vi "test13-AsteriskWildcardStateRegistration.vi"(8 "error in (no error)":errorcluster, 11 "TestCase in":refnum<class "testcase-CSMBroadcast.lvclass">) -> (0 "error out":errorcluster, 3 "TestCase out":refnum<class "testcase-CSMBroadcast.lvclass">)   [LabVIEW 2017, in "testcase-CSMBroadcast.lvclass"]
uses:
  testcase-CSMBroadcast.lvclass
  0c20cacf-7d77-4f8e-aec5-f22e7d09936d.vi
  26de337d-8090-412f-9da5-e117a55d4726.vi
  de10340a-d592-45ad-b055-7fa7b377c551.vi
  e3eae2f8-d8ce-4adb-8167-9a417250fce1.vi
  a4d00e00-a9ed-4631-bf53-269bf71f16fc.vi
  src/user.lib/_NEVSTOP/Communicable State Machine(CSM)/AdvanceAPI/CSM - Revert Arguments-Safe String.vi
  src/user.lib/_NEVSTOP/Communicable State Machine(CSM)/_Shared/Trim Single-line Text.vi
  src/user.lib/_NEVSTOP/Communicable State Machine(CSM)/AdvanceAPI/CSM - Make String Arguments Safe.vi
  src/user.lib/_NEVSTOP/Communicable State Machine(CSM)/AdvanceAPI/CSM - Break Down Multiple States String.vi
  src/user.lib/_NEVSTOP/Communicable State Machine(CSM)/AdvanceAPI/CSM - Compact Multiple States.vi
  src/user.lib/_NEVSTOP/Communicable State Machine(CSM)/AdvanceAPI/CSM - Keywords.vi
  src/user.lib/_NEVSTOP/Communicable State Machine(CSM)/AdvanceAPI/CSM - Set Module Attribute.vi
  src/user.lib/_NEVSTOP/Communicable State Machine(CSM)/AdvanceAPI/CSM - Get Module Attribute.vi
  <vilib>/addons/_JKI Toolkits/VI Tester/TestCase.llb/TestCase.lvclass
  src/user.lib/_NEVSTOP/Communicable State Machine(CSM)/Communicable State Machine.lvlib
  C:/Program Files (x86)/National Instruments/LabVIEW 2017/vi.lib/addons/_JKI Toolkits/VI Tester/TestCase.llb/TestCase.lvclass
panel:
  out "Execution Times":i32
  out "State History":string
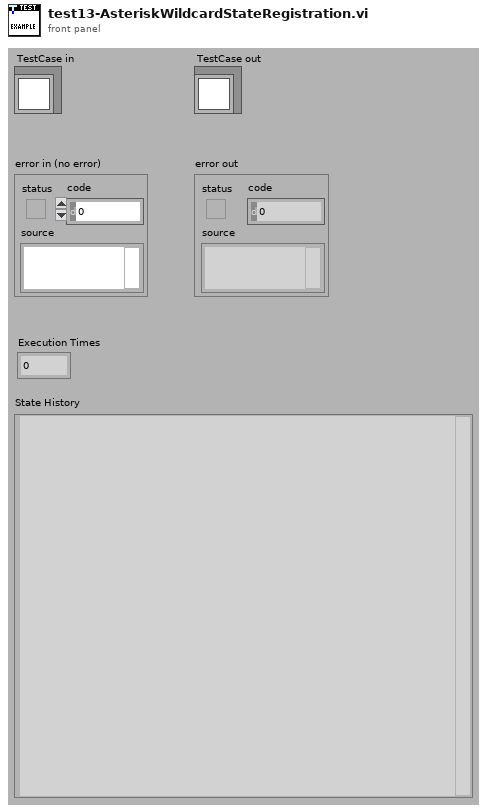
[diagram p1: front panel]
types:
  T1 = enum32{"Invalid", "Standard", "Closed", "Hidden", "Minimized", "Maximized"}
  T2 = enum32{"invalid app kind", "Development System", "Run Time System", "Student Edition", "Embedded LabVIEW", "Evaluation", "Custom"}
  T3 = typedef "Communicable State Machine.lvlib/_CSM_Response Source Message.ctl" = cluster{"‘State":string, "’Arguments":string, "’Error":errorcluster}
  T4 = cluster{"Current VI Reference":refnum<vi>, "Close Panel on Exit?":bool}
  T5 = cluster{"Core":cluster{"Current VI Reference":refnum<vi>, "Close Panel on Exit?":bool}, "Your Boolean data":bool, "Your string data":string, "TestData":i32}
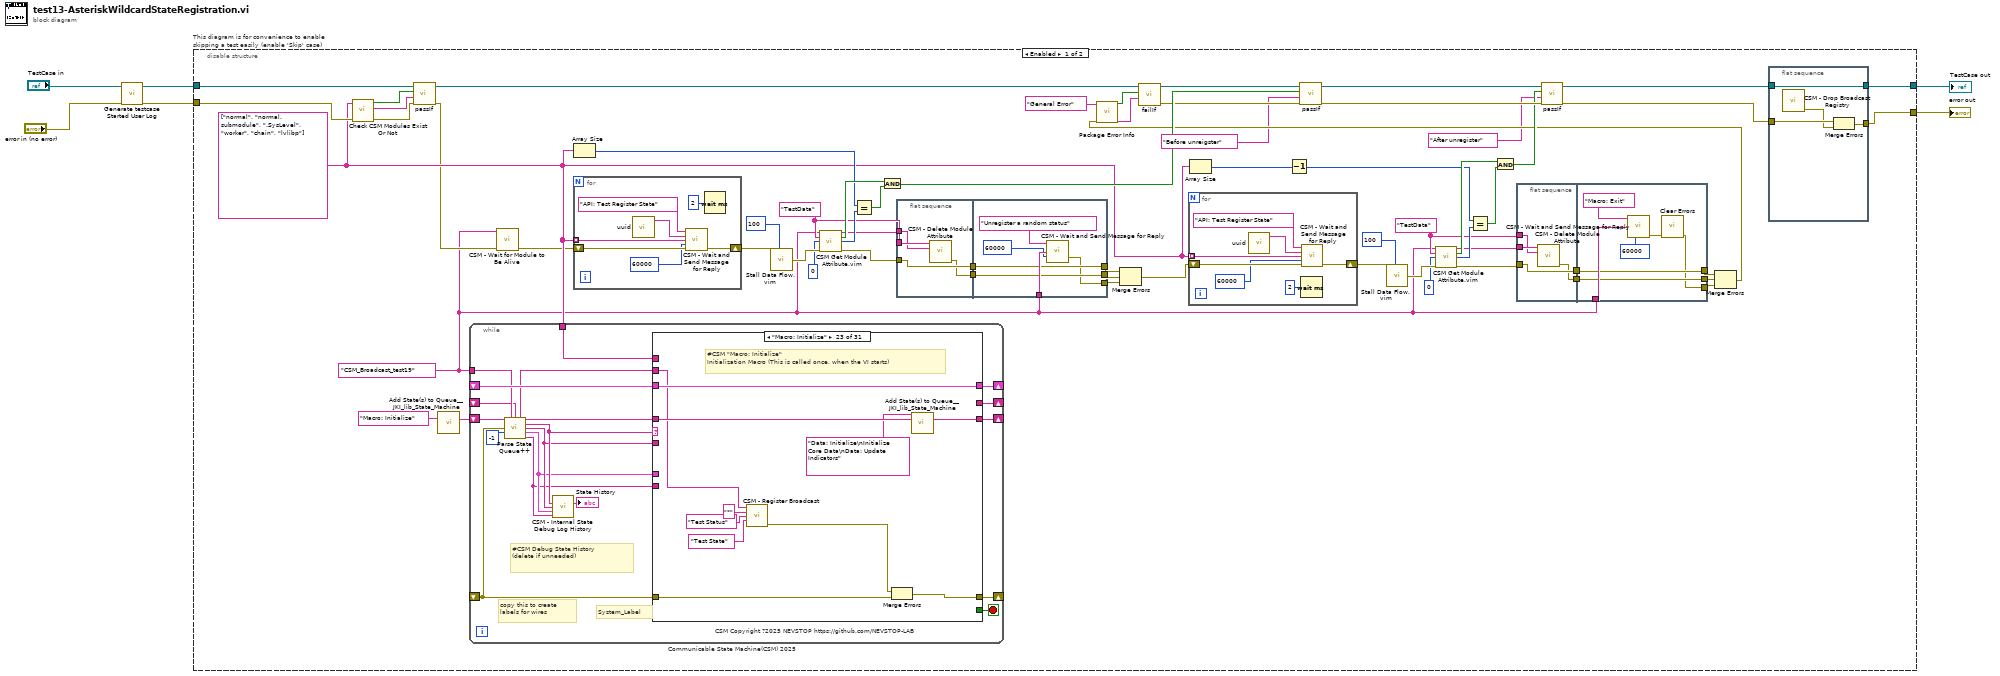
[diagram p0: block diagram]
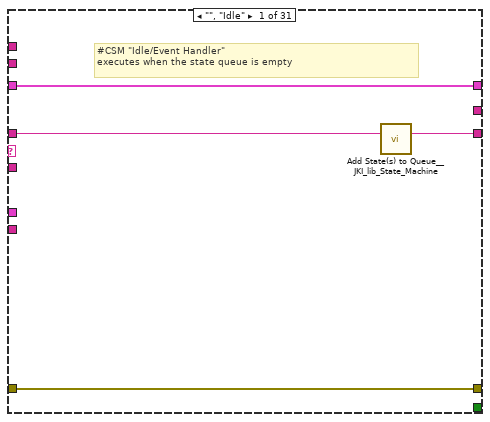
[diagram p2: hidden frame]
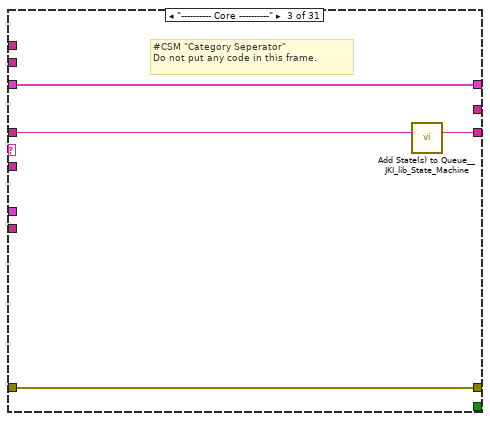
[diagram p4: hidden frame]
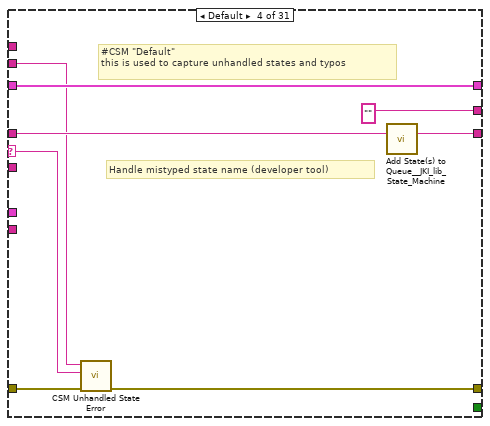
[diagram p5: hidden frame]
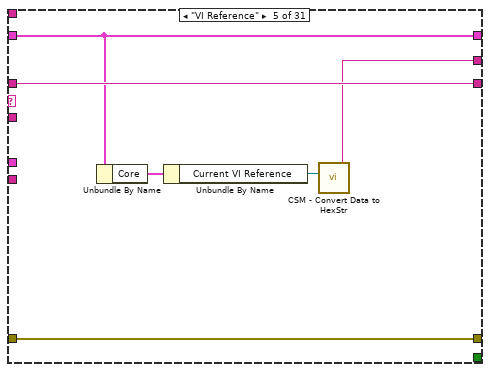
[diagram p6: hidden frame]
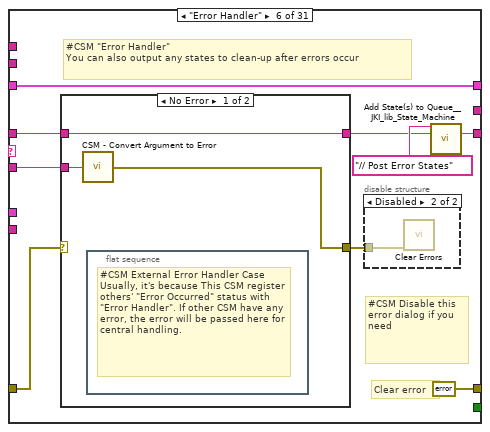
[diagram p7: hidden frame]
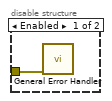
[diagram p8: hidden frame]
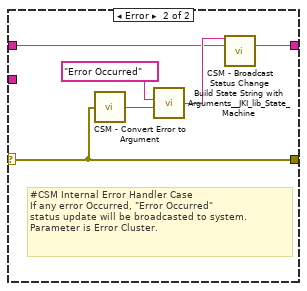
[diagram p9: hidden frame]
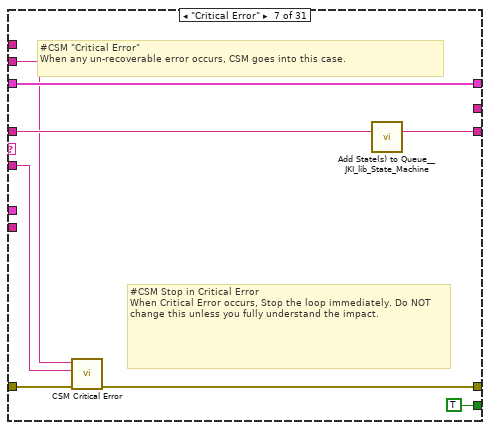
[diagram p10: hidden frame]
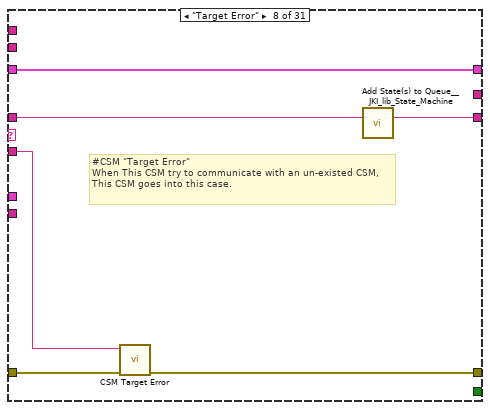
[diagram p11: hidden frame]
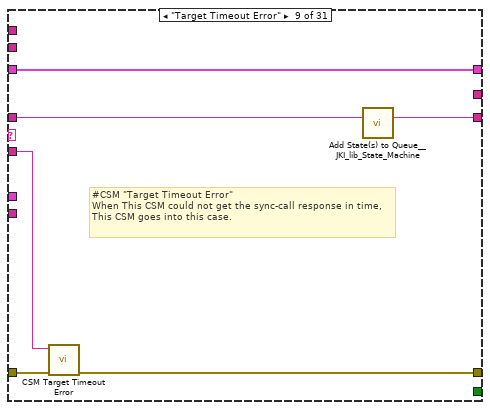
[diagram p12: hidden frame]
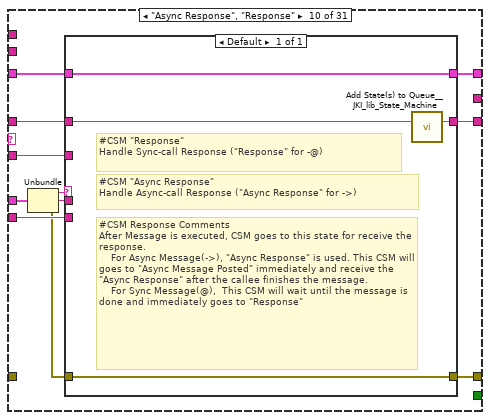
[diagram p13: hidden frame]
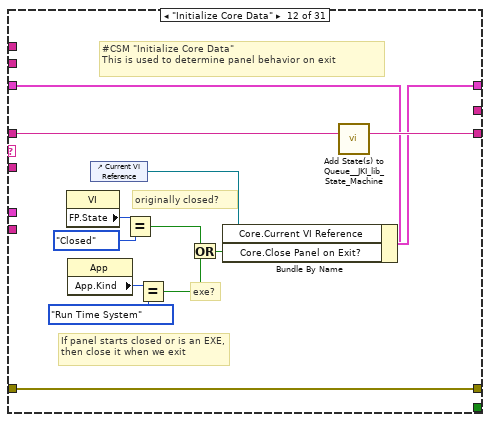
[diagram p15: hidden frame]
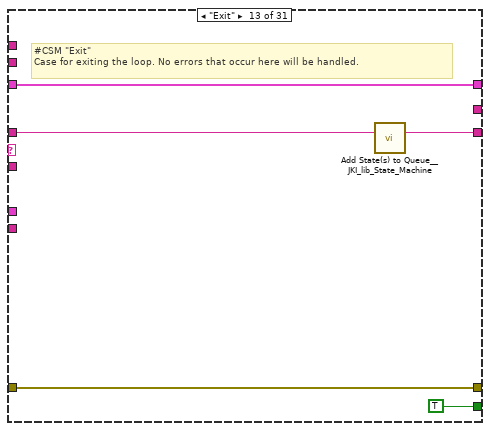
[diagram p16: hidden frame]
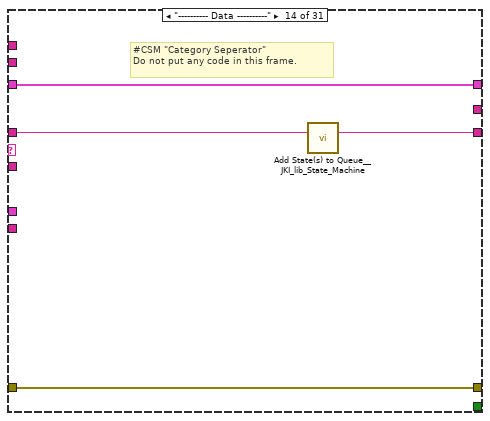
[diagram p17: hidden frame]
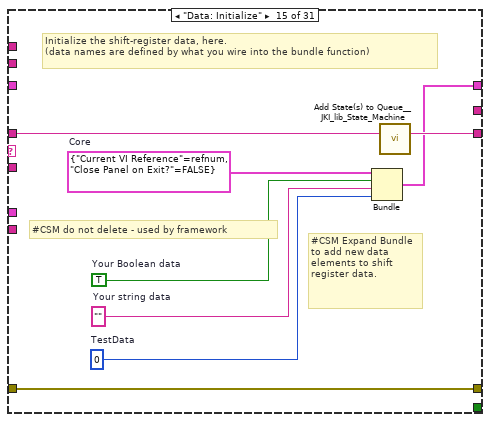
[diagram p18: hidden frame]
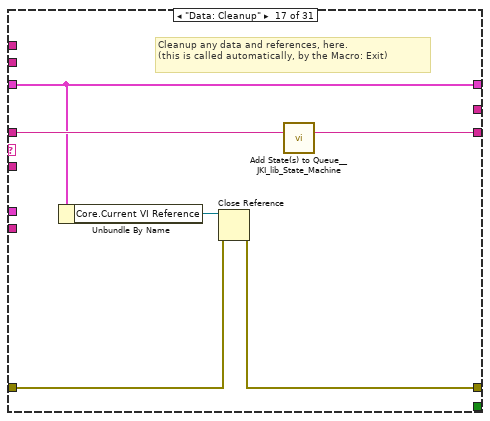
[diagram p20: hidden frame]
diagram:
  n1 = call "Generate testcase Started User Log.vi"("Error In"="error in (no error)") -> ("error out"=w1:errorcluster)  [unwired: 10 in]
  n2 = disable-structure "This diagram is for convenience to enable skipping a test easily (enable 'Skip' case)" shown="Enabled" {
    disable-tunnel: "TestCase in" -> [w24 w426]
    disable-tunnel: [w19 w424] -> w2
    disable-tunnel: [w18 w425] -> w4
    disable-tunnel: w1 -> [w23 w423]
    frame Enabled {
      w33 = "TestData" ("Attribute")
      w55 = "TestData" ("Attribute")
      w6 = "CSM_Broadcast_test19" ("Name (\"\" to Use UUID)")
      w22 = string[] ["normal", "normal.submodule", ".SysLevel", "worker", "chain", "lvlibp"]
      n3 = call "Check CSM Modules Exist Or Not.vi"("error in"=w23, "CSM names in"=w22) -> ("error out"=w25:errorcluster, "Debug string"=w26:string, "All Modules Exist?"=w27:bool)  [unwired: 7 in]
      n4 = call-dynamic "passIf.vi"("error in (no error)"=w25, "message (\"\")"=w26, "pass"=w27, "TestCase in"=w24) -> ("error out"=w7:errorcluster, "TestCase out"=w16:refnum<class "testcase-CSMBroadcast.lvclass">)  [unwired: 6 in]
      n5 = call <vilib>:"Add State(s) to Queue__JKI_lib_State_Machine.vi"("State(s) in (\"\")"="Macro: Initialize" ("Init State(\"Macro: Initialize\")")) -> ("States Out"=w66:string)  [unwired: 14 in]
      n6 = while "Communicable State Machine(CSM) 2025" {
        shift-right: [w113] -> _
        shift-left: _ -> [w112]
        shift-right: [w116] -> _
        shift-left: _ -> [w111]
        shift-right: [w115] -> _
        shift-left: w66 -> [w117]
        tunnel: w6 -> [w109]
        shift-right: [w110] -> _
        shift-left: _ -> [w103]
        tunnel: w22 -> [w100]
        stop <- w114 stop-if-true
        # "#CSM Debug State History\n(delete if unneeded)"
        # "copy this to create labels for wires"
        # "System_Label"
        # "CSM Copyright ?2025 NEVSTOP https://github.com/NEVSTOP-LAB"
        n7 = call "Parse State Queue++.vi"("State Queue"=w117, "Name (\"\" to Use UUID)"=w109, "Response Arguments"=w103, "Previous Error"=w111, "Dequeue (1 ms)"=-1 ("Timeout")) -> ("Name Used"=w104:string, "Remaining States"=w118:string, "Current State"=w108:string, "Arguments"=w107:string, "Additional Information"=w106:T3, "Source CSM"=w105:string)  [unwired: 5 in]
        n8 = call "CSM - Internal State Debug Log History.vi"("State"=w108, "Arguments (\"\")"=w107, ">> Response Source Message >>"=w106, "Source (\"\")"=w105) -> ("Debug Log"=→"State History":string)  [unwired: 11 in]
        n9 = case shown="\"Macro: Initialize\"" w108 {
          selector: w108 -> [_ _ _ w132 _ _ _ _ _ _ _ _ _ _ _ _ _ _ _ _ _ _ _ _ _ _ _ _ _ _ _]
          tunnel: w118 -> [w119 w124 w129 w136 w142 w148 w169 w175 w181 w189 w200 w214 w219 w223 w231 w233 w240 w244 w248 w254 w269 w338 w349 w362 w364 w368 w373 w380 w384 w395 w415]
          tunnel: w107 -> [_ _ _ _ _ w147 w165 w174 w179 w188 _ _ _ _ _ _ _ _ _ w249 w263 _ _ _ _ _ w371 _ _ _ _]
          tunnel: w112 -> [w120 w123 w126 w134 w141 w151 w170 w176 w182 w191 w199 w207 w217 w220 _ w232 w235 w241 w246 w252 w265 w335 w346 w359 w363 w367 w372 w377 w381 w387 w401]
          tunnel: [w121 w125 w127 w130 w143 errorcluster {"status"=FALSE, "code"=0, "source"=""} ("error out") w166 w172 w178 w194 w201 w211 w216 w221 w228 w234 w236 w242 w245 w250 w266 w336 w340 w351 w365 w369 w374 w378 w382 w389 w403] -> w116
          tunnel: w111 -> [w121 w125 w127 w137 w143 w149 w171 w173 w180 _ w201 w211 w216 w221 w228 w234 w237 w242 w245 w251 w267 w336 w347 w360 w365 w369 w374 w378 w382 w393 w413]
          tunnel: [w122 w124 w128 w135 w142 w144 w168 w177 w183 w190 w200 w213 w218 w222 w230 w233 w239 w243 w247 w253 w268 w337 w348 w361 w364 w368 w373 w379 w383 w394 w414] -> w115
          tunnel: [_ _ _ _ _ _ TRUE _ _ _ _ _ TRUE _ _ _ _ _ _ _ _ _ _ _ _ _ _ _ _ _ _] -> w114
          tunnel: [w120 w123 w126 w134 w141 w151 w170 w176 w182 w192 w199 w212 w217 w220 w229 w232 w235 w241 w246 w252 w265 w335 w346 w359 w363 w367 w372 w377 w381 w391 w399] -> w113
          tunnel: w105 -> [_ _ _ _ _ _ _ _ _ w186 _ _ _ _ _ _ _ _ _ _ _ _ _ _ _ _ _ _ _ _ _]
          tunnel: w106 -> [_ _ _ _ _ _ _ _ _ w193 _ _ _ _ _ _ _ _ _ _ _ _ _ _ _ _ _ _ _ _ _]
          tunnel: [_ _ _ "" w138 _ _ _ _ _ _ _ _ _ _ _ _ _ _ _ _ _ _ _ _ "API1 Response" w370 _ _ _ _] -> w110
          tunnel: w104 -> [_ _ _ w131 _ _ w164 _ _ _ _ _ _ _ _ _ _ _ _ _ _ _ w341 w353 _ _ _ _ _ w390 w410]
          tunnel: w100 -> [_ _ _ _ _ _ _ _ _ _ _ _ _ _ _ _ _ _ _ _ _ _ _ _ _ _ _ _ _ _ w406]
          frame "", "Idle" {
            # "#CSM \"Idle/Event Handler\"\nexecutes when the state queue is empty"
            n10 = call <vilib>:"Add State(s) to Queue__JKI_lib_State_Machine.vi"("State(s) in (\"\")"=w119) -> ("States Out"=w122:string)  [unwired: 14 in]
          }
          frame "CSM Documentation" {
            # "#CSM README FIRST\n\nCommunicable State Machine(CSM) is a LabVIEW application framework that builds upon JKI State Machine(JKISM). It follows the pattern of JKISM and extends the keywords to describe message communication between modules, including concepts such as Sync-Message, Async-Message, Subscription/Unsubscription of status - essential elements for creating reusable code modules. For more information, please visit the CSM wiki: https://nevstop-lab.github.io/CSM-Wiki/\n\nFor instructions on JKI State Machine, visit: http://jki.net/state-machine/\nFor information about CSM, visit: https://github.com/NEVSTOP-LAB"
            # "#CSM \"Documentation\"\nCase for holding CSM Documenation"
          }
          frame "---------- Core ----------" {
            # "#CSM \"Category Seperator\"\nDo not put any code in this frame."
            n11 = call <vilib>:"Add State(s) to Queue__JKI_lib_State_Machine.vi"("State(s) in (\"\")"=w129) -> ("States Out"=w128:string)  [unwired: 14 in]
          }
          frame Default {
            # "#CSM \"Default\"\nthis is used to capture unhandled states and typos"
            # "Handle mistyped state name (developer tool)"
            n12 = call "CSM Unhandled State Error.vi"("error in (no error)"=w137, "Undefined State"=w132, "CSM Name"=w131) -> ("error out"=w130:errorcluster)  [unwired: 8 in]
            n13 = call <vilib>:"Add State(s) to Queue__JKI_lib_State_Machine.vi"("State(s) in (\"\")"=w136) -> ("States Out"=w135:string)  [unwired: 14 in]
          }
          frame "VI Reference" {
            n14 = Unbundle By Name(w141) -> ("Core"=w140:T4)
            n15 = Unbundle By Name(w140) -> ("Current VI Reference"=w139:refnum<vi>)
            n16 = call "CSM - Convert Data to HexStr.vi"("Variant"=w139) -> ("HEX String (0-9,A-F)"=w138:string)  [unwired: 8 in]
          }
          frame "Error Handler" {
            # "#CSM Disable this error dialog if you need"
            # "#CSM \"Error Handler\"\nYou can also output any states to clean-up after errors occur"
            # "Clear error"
            n17 = case shown="No Error" w149 {
              selector: w149 -> [_ w158]
              tunnel: [w157 w160] -> w145
              tunnel: w148 -> [w157 w159]
              tunnel: w147 -> [w156 _]
              tunnel: [w155 w158] -> w150
              frame No Error {
                n18 = call "CSM - Convert Argument to Error.vi"("Argument"=w156) -> ("Error"=w155:errorcluster)  [unwired: 4 in]
                n19 = flat-sequence {
                  frame #0 {
                    # "#CSM External Error Handler Case\nUsually, it's because This CSM register others' \"Error Occurred\" status with \"Error Handler\". If other CSM have any error, the error will be passed here for central handling."
                  }
                }
              }
              frame Error {
                # "#CSM Internal Error Handler Case \nIf any error Occurred, \"Error Occurred\" \nstatus update will be broadcasted to system.\nParameter is Error Cluster."
                n20 = call "CSM - Convert Error to Argument.vi"("Error"=w158) -> ("Argument"=w162:string)  [unwired: 4 in]
                n21 = call <vilib>:"Build State String with Arguments__JKI_lib_State_Machine.vi"("Arguments (\"\")"=w162, "State"="Error Occurred" ("Status with Arguments")) -> ("State with Arguments"=w161:string)  [unwired: 4 in]
                n22 = call "CSM - Broadcast Status Change.vi"("Status With Arguments"=w161, "State Queue"=w159) -> ("Remaining States"=w160:string)  [unwired: 13 in]
              }
            }
            n23 = disable-structure shown="Disabled" {
              disable-tunnel: w150 -> [w153 w154]
              frame Enabled {
                n24 = call <vilib>:"General Error Handler.vi"("error in (no error)"=w153) -> ()  [unwired: 10 in, 5 out]
              }
              frame Disabled {
                n25 = call <vilib>:"Clear Errors.vi"("error in (no error)"=w154) -> ()  [unwired: 5 in, 2 out]
              }
            }
            n26 = call <vilib>:"Add State(s) to Queue__JKI_lib_State_Machine.vi"("State(s) in Front (\"\")"="// Post Error States", "State(s) in (\"\")"=w145) -> ("States Out"=w144:string)  [unwired: 13 in]
          }
          frame "Critical Error" {
            # "#CSM Stop in Critical Error\nWhen Critical Error occurs, Stop the loop immediately. Do NOT change this unless you fully understand the impact."
            # "#CSM \"Critical Error\"\nWhen any un-recoverable error occurs, CSM goes into this case."
            n27 = call "CSM Critical Error.vi"("error in (no error)"=w171, "Arugments (As Reason)"=w165, "CSM Name"=w164) -> ("error out"=w166:errorcluster)  [unwired: 8 in]
            n28 = call <vilib>:"Add State(s) to Queue__JKI_lib_State_Machine.vi"("State(s) in (\"\")"=w169) -> ("States Out"=w168:string)  [unwired: 14 in]
          }
          frame "Target Error" {
            # "#CSM \"Target Error\"\nWhen This CSM try to communicate with an un-existed CSM, This CSM goes into this case."
            n29 = call "CSM Target Error.vi"("error in (no error)"=w173, "Arguments (As CSM Name)"=w174) -> ("error out"=w172:errorcluster)  [unwired: 9 in]
            n30 = call <vilib>:"Add State(s) to Queue__JKI_lib_State_Machine.vi"("State(s) in (\"\")"=w175) -> ("States Out"=w177:string)  [unwired: 14 in]
          }
          frame "Target Timeout Error" {
            # "#CSM \"Target Timeout Error\"\nWhen This CSM could not get the sync-call response in time, This CSM goes into this case."
            n31 = call "CSM Target Timeout Error.vi"("error in (no error)"=w180, "Arguments (As CSM Name)"=w179) -> ("error out"=w178:errorcluster)  [unwired: 9 in]
            n32 = call <vilib>:"Add State(s) to Queue__JKI_lib_State_Machine.vi"("State(s) in (\"\")"=w181) -> ("States Out"=w183:string)  [unwired: 14 in]
          }
          frame "Async Response", "Response" {
            n33 = Unbundle(w193) -> ("‘State"=w187:string, "’Arguments"=w185:string, "’Error"=w184:errorcluster)
            n34 = case shown="Default" w187 {
              tunnel: [w198] -> w194
              tunnel: w184 -> [w198]
              tunnel: [w197] -> w192
              tunnel: w191 -> [w197]
              tunnel: [w195] -> w190
              tunnel: w189 -> [w196]
              tunnel: w188 -> [_]
              tunnel: w186 -> [_]
              tunnel: w185 -> [_]
              frame Default {
                # "#CSM Response Comments\nAfter Message is executed, CSM goes to this state for receive the response.\n    For Async Message(->), \"Async Response\" is used. This CSM will goes to \"Async Message Posted\" immediately and receive the \"Async Response\" after the callee finishes the message.\n    For Sync Message(@),  This CSM will wait until the message is done and immediately goes to \"Response\""
                # "#CSM \"Async Response\"\nHandle Async-call Response (\"Async Response\" for ->)"
                # "#CSM \"Response\"\nHandle Sync-call Response (\"Response\" for -@)"
                n35 = call <vilib>:"Add State(s) to Queue__JKI_lib_State_Machine.vi"("State(s) in (\"\")"=w196) -> ("States Out"=w195:string)  [unwired: 14 in]
              }
            }
          }
          frame "Async Message Posted" {
            # "#CSM \"Async Message Posted\"\nAfter Async Message is posted (-> or ->| ), CSM goes to this state for post-action.\nYou can use Argument - State to tell which Async Message is called."
          }
          frame "Initialize Core Data" {
            # "#CSM \"Initialize Core Data\"\nThis is used to determine panel behavior on exit"
            # "originally closed?"
            # "exe?"
            # "If panel starts closed or is an EXE, then close it when we exit"
            n36 = property class="VI"() -> ("FP.State"=w204:T1)  [unwired: 2 in, 2 out]
            n37 = property class="App"() -> ("App.Kind"=w210:T2)  [unwired: 2 in, 2 out]
            n38 = control-ref of="Current VI Reference"() -> (w205:refnum<vi>)
            n39 = Equal?(x=w204, y=T1."Closed" ("Front Panel Window:State")) -> (x = y?=w202:bool)
            n40 = Equal?(x=w210, y=T2."Run Time System" ("Application:Kind")) -> (x = y?=w208:bool)
            n41 = Or(x=w202, y=w208) -> (x .or. y?=w206:bool)
            n42 = Bundle By Name(cluster=w207, "Core.Current VI Reference"=w205, "Core.Close Panel on Exit?"=w206) -> (w212:T5)
            n43 = call <vilib>:"Add State(s) to Queue__JKI_lib_State_Machine.vi"("State(s) in (\"\")"=w214) -> ("States Out"=w213:string)  [unwired: 14 in]
          }
          frame "Exit" {
            # "#CSM \"Exit\"\nCase for exiting the loop. No errors that occur here will be handled."
            n44 = call <vilib>:"Add State(s) to Queue__JKI_lib_State_Machine.vi"("State(s) in (\"\")"=w219) -> ("States Out"=w218:string)  [unwired: 14 in]
          }
          frame "---------- Data ----------" {
            # "#CSM \"Category Seperator\"\nDo not put any code in this frame."
            n45 = call <vilib>:"Add State(s) to Queue__JKI_lib_State_Machine.vi"("State(s) in (\"\")"=w223) -> ("States Out"=w222:string)  [unwired: 14 in]
          }
          frame "Data: Initialize" {
            w224 = 0  # TestData
            w225 = T4 {"Current VI Reference"=refnum, "Close Panel on Exit?"=FALSE}  # Core
            w227 = TRUE  # Your Boolean data
            w226 = ""  # Your string data
            # "#CSM do not delete - used by framework"
            # "#CSM Expand Bundle to add new data elements to shift register data."
            # "Initialize the shift-register data, here.\n(data names are defined by what you wire into the bundle function)"
            n46 = Bundle("Core"=w225, "Your Boolean data"=w227, "Your string data"=w226, "TestData"=w224) -> (w229:T5)  [unwired: 1 in]
            n47 = call <vilib>:"Add State(s) to Queue__JKI_lib_State_Machine.vi"("State(s) in (\"\")"=w231) -> ("States Out"=w230:string)  [unwired: 14 in]
          }
          frame "Data: Update Indicators" {
          }
          frame "Data: Cleanup" {
            # "Cleanup any data and references, here.\n(this is called automatically, by the Macro: Exit)"
            n48 = Unbundle By Name(w235) -> ("Core.Current VI Reference"=w238:refnum<vi>)
            n49 = Close Reference(reference=w238, error in (no error)=w237) -> (error out=w236:errorcluster)
            n50 = call <vilib>:"Add State(s) to Queue__JKI_lib_State_Machine.vi"("State(s) in (\"\")"=w240) -> ("States Out"=w239:string)  [unwired: 14 in]
          }
          frame "---------- UI ----------" {
            # "#CSM \"Category Seperator\"\nDo not put any code in this frame."
            n51 = call <vilib>:"Add State(s) to Queue__JKI_lib_State_Machine.vi"("State(s) in (\"\")"=w244) -> ("States Out"=w243:string)  [unwired: 14 in]
          }
          frame "UI: Initialize" {
            # "#CSM \"UI: Initialize\"\nInitialize the User Interface, here.\n(this is called automatically, by the Macro: Init)"
            n52 = call <vilib>:"Add State(s) to Queue__JKI_lib_State_Machine.vi"("State(s) in (\"\")"=w248) -> ("States Out"=w247:string)  [unwired: 14 in]
          }
          frame "UI: Cursor Set" {
            # "#CSM \"UI: Cursor Set\"\nSet and Unset Cursor Busy.\n(Usage: \"UI: Cursor Set >> Busy|Idle\")"
            # "Argument"
            n53 = disable-structure shown="TARGET_TYPE!=Windows" {
              disable-tunnel: w251 -> [w257 w262]
              disable-tunnel: [w256 w262] -> w250
              disable-tunnel: w249 -> [w255 _]
              frame condition #0 (active) {
                n54 = case shown="\"Idle\", Default" w255 {
                  tunnel: w257 -> [w259 w261]
                  tunnel: [w258 w260] -> w256
                  frame "Idle", Default {
                    n55 = call <vilib>:"Unset Busy.vi"("error in (no error)"=w259) -> ("error out"=w258:errorcluster)  [unwired: 10 in]
                  }
                  frame "Busy" {
                    n56 = call <vilib>:"Set Busy.vi"("error in (no error)"=w261) -> ("error out"=w260:errorcluster)  [unwired: 9 in, 1 out]
                  }
                }
              }
              frame condition #1 {
              }
            }
            n57 = call <vilib>:"Add State(s) to Queue__JKI_lib_State_Machine.vi"("State(s) in (\"\")"=w254) -> ("States Out"=w253:string)  [unwired: 14 in]
          }
          frame "UI: Front Panel State" {
            # "#CSM \"UI: Front Panel State\"\nSet Front Panel Open or Closed\n(Usage: \"UI: Front Panel State >> Open|Close\")"
            # "Argument"
            n58 = Unbundle By Name(w265) -> ("Core.Current VI Reference"=w264:refnum<vi>)
            n59 = call <vilib>:"Add State(s) to Queue__JKI_lib_State_Machine.vi"("State(s) in (\"\")"=w269) -> ("States Out"=w268:string)  [unwired: 14 in]
            n60 = case shown="\"Close\", \"Closed\"" w263 {
              tunnel: w267 -> [w275 w290 w301 w314 w327]
              tunnel: [w277 w291 w303 w316 w329] -> w266
              tunnel: w264 -> [w276 w288 w302 w315 w328]
              frame "Open", "Standard", Default {
                w270 = T1."Standard" ("State")
                n61 = property class="VI"(reference=w276, error in=w275) -> (reference out=w273:refnum<vi>, error out=w274:errorcluster, "FP.State"=w272:T1)
                n62 = Not Equal?(x=w272, y=w270) -> (x != y?=w271:bool)
                n63 = case shown="True" w271 {
                  tunnel: [w281 w283] -> w277
                  tunnel: w274 -> [w280 w283]
                  tunnel: w273 -> [w279 _]
                  tunnel: w270 -> [w278 _]
                  frame True {
                    n64 = invoke class="VI" method="FP.Open"(reference=w279, error in=w280, "Activate"=TRUE, "State"=w278) -> (error out=w281:errorcluster)  [unwired: 1 in, 4 out]
                  }
                  frame False {
                  }
                }
              }
              frame "Close", "Closed" {
                n65 = property class="VI"(reference=w288, error in=w290) -> (reference out=w287:refnum<vi>, error out=w289:errorcluster, "FP.State"=w285:T1)
                n66 = Not Equal?(x=w285, y=T1."Closed" ("Front Panel Window:State")) -> (x != y?=w284:bool)
                n67 = case shown="False" w284 {
                  tunnel: [w292 w295] -> w291
                  tunnel: w289 -> [w292 w294]
                  tunnel: w287 -> [_ w293]
                  frame False {
                  }
                  frame True {
                    n68 = invoke class="VI" method="FP.Close"(reference=w293, error in=w294) -> (error out=w295:errorcluster)  [unwired: 1 in, 2 out]
                  }
                }
              }
              frame "Hidden", "Hide" {
                w296 = T1."Hidden" ("State")
                n69 = property class="VI"(reference=w302, error in=w301) -> (reference out=w299:refnum<vi>, error out=w300:errorcluster, "FP.State"=w298:T1)
                n70 = Not Equal?(x=w298, y=w296) -> (x != y?=w297:bool)
                n71 = case shown="True" w297 {
                  tunnel: [w307 w308] -> w303
                  tunnel: w300 -> [w306 w308]
                  tunnel: w299 -> [w305 _]
                  tunnel: w296 -> [w304 _]
                  frame True {
                    n72 = invoke class="VI" method="FP.Open"(reference=w305, error in=w306, "State"=w304) -> (error out=w307:errorcluster)  [unwired: 2 in, 4 out]
                  }
                  frame False {
                  }
                }
              }
              frame "Minimize", "Minimized" {
                w309 = T1."Minimized" ("State")
                n73 = property class="VI"(reference=w315, error in=w314) -> (reference out=w312:refnum<vi>, error out=w313:errorcluster, "FP.State"=w311:T1)
                n74 = Not Equal?(x=w311, y=w309) -> (x != y?=w310:bool)
                n75 = case shown="True" w310 {
                  tunnel: [w320 w321] -> w316
                  tunnel: w313 -> [w319 w321]
                  tunnel: w312 -> [w318 _]
                  tunnel: w309 -> [w317 _]
                  frame True {
                    n76 = invoke class="VI" method="FP.Open"(reference=w318, error in=w319, "State"=w317) -> (error out=w320:errorcluster)  [unwired: 2 in, 4 out]
                  }
                  frame False {
                  }
                }
              }
              frame "Maximize", "Maximized" {
                w322 = T1."Maximized" ("State")
                n77 = property class="VI"(reference=w328, error in=w327) -> (reference out=w325:refnum<vi>, error out=w326:errorcluster, "FP.State"=w324:T1)
                n78 = Not Equal?(x=w324, y=w322) -> (x != y?=w323:bool)
                n79 = case shown="True" w323 {
                  tunnel: [w333 w334] -> w329
                  tunnel: w326 -> [w332 w334]
                  tunnel: w325 -> [w331 _]
                  tunnel: w322 -> [w330 _]
                  frame True {
                    n80 = invoke class="VI" method="FP.Open"(reference=w331, error in=w332, "State"=w330) -> (error out=w333:errorcluster)  [unwired: 2 in, 4 out]
                  }
                  frame False {
                  }
                }
              }
            }
          }
          frame "---------- Macro ----------" {
            # "#CSM \"Category Seperator\"\nDo not put any code in this frame."
            n81 = call <vilib>:"Add State(s) to Queue__JKI_lib_State_Machine.vi"("State(s) in (\"\")"=w338) -> ("States Out"=w337:string)  [unwired: 14 in]
          }
          frame "Macro: Initialize" {
            # "#CSM \"Macro: Initialize\"\nInitialization Macro (This is called once, when the VI starts)"
            n82 = call "CSM - Register Broadcast.vi"("CSM Name(Empty for Broadcast Event)"=w341, "Source CSM Name (* as Default)"="*", "Trigger"="Test Status" ("Status"), "API (If \"\", Same as Trigger)"="Test State" ("Response Message (If \"\", Same as Source Message)")) -> ("error out"=w339:errorcluster)  [unwired: 10 in, 1 out]
            n83 = Merge Errors(w339, w347) -> (w340:errorcluster)
            n84 = call <vilib>:"Add State(s) to Queue__JKI_lib_State_Machine.vi"("State(s) in Front (\"\")"="Data: Initialize\nInitialize Core Data\nData: Update Indicators", "State(s) in (\"\")"=w349) -> ("States Out"=w348:string)  [unwired: 13 in]
          }
          frame "Macro: Exit" {
            # "#CSM \"Macro: Exit\"\nExit Macro (This is called once, when the VI exits)"
            n85 = call "CSM - Unregister Broadcast.vi"("CSM Name(Empty for Broadcast Event)"=w353, "Source CSM Name (* as Default)"="*", "Trigger"="Test Status" ("Status"), "API (\"*\" as Default)"="Test State" ("Response Message (If \"\", Same as Source Message)")) -> ("error out"=w350:errorcluster)  [unwired: 10 in, 1 out]
            n86 = call <vilib>:"Add State(s) to Queue__JKI_lib_State_Machine.vi"("State(s) in Front (\"\")"="//Exit Sub-Modules ", "State(s) at Back (\"\")"="Data: Cleanup\nExit") -> ("States Out"=w357:string)  [unwired: 13 in]
            n87 = Merge Errors(w350, w360) -> (w351:errorcluster)
            n88 = call <vilib>:"Add State(s) to Queue__JKI_lib_State_Machine.vi"("State(s) in Front (\"\")"=w357, "State(s) in (\"\")"=w362) -> ("States Out"=w361:string)  [unwired: 13 in]
          }
          frame "---------- API ----------" {
            # "#CSM \"Category Seperator\"\nDo not put any code in this frame."
          }
          frame "API: API1" {
            # "#CSM API Example\nCopy/Rename this case for your own API"
            # "#CSM Response\nConnect this to return the response of your API"
            # "#CSM >> Msg/Rep's CSM >>\nIf you need to tell who triggered this state , use this string. If it's this case itself, this string is \"\"."
            # "#CSM >> Arguments >>\nDeal with the parameter if any"
          }
          frame "API: API2" {
            # "#CSM API Example\nCopy/Rename this case for your own API"
            # "unpack Hex String  to Variant\nif complex parameter is needed."
            n89 = call "CSM - Convert HexStr to Data.vi"("HEX String"=w371) -> ()  [unwired: 7 in, 2 out]
            n90 = disable-structure shown="Disabled" {
              disable-tunnel: [w375 "API2 Response"] -> w370
              frame Disabled {
                # "pack variant to hexstr \nif complex response is needed."
                # "complex Response"
                n91 = call "CSM - Convert Data to HexStr.vi"() -> ("HEX String (0-9,A-F)"=w375:string)  [unwired: 9 in]
              }
              frame Enabled {
              }
            }
          }
          frame "---------- Action ----------" {
            # "#CSM \"Category Seperator\"\nDo not put any code in this frame."
            n92 = call <vilib>:"Add State(s) to Queue__JKI_lib_State_Machine.vi"("State(s) in (\"\")"=w380) -> ("States Out"=w379:string)  [unwired: 14 in]
          }
          frame "Action: action1" {
            # "#CSM \"Internal State\"\nThis category is used for holding internal states"
            n93 = call <vilib>:"Add State(s) to Queue__JKI_lib_State_Machine.vi"("State(s) in (\"\")"=w384) -> ("States Out"=w383:string)  [unwired: 14 in]
          }
          frame "Test State" {
            n94 = Unbundle By Name(w387) -> ("TestData"=w392:i32)
            n95 = disable-structure shown="Enabled" {
              frame Disabled {
                n96 = feedback #1(0 ("y")) -> (w397:i32)
                n97 = Increment(x=w397) -> (x+1=w396:i32)
                "Execution Times" <- w396
                n98 = feedback-in #1(w396) -> ()
              }
              frame Enabled {
              }
            }
            n99 = Increment(x=w392) -> (x+1=w385:i32)
            n100 = Bundle By Name(cluster=w387, "TestData"=w385) -> (w391:T5)
            n101 = call "CSM Set Module Attribute.vim"("CSM Name"=w390, "Attribute"="TestData", "Value"=w385) -> ("error out"=w388:errorcluster)  [unwired: 9 in, 3 out]
            n102 = call <vilib>:"Add State(s) to Queue__JKI_lib_State_Machine.vi"("State(s) in (\"\")"=w395) -> ("States Out"=w394:string)  [unwired: 14 in]
            n103 = Merge Errors(w393, w388) -> (w389:errorcluster)
          }
          frame "Unregister a random status" {
            n104 = Random Number (0-1)() -> (number: 0 to 1=w408:dbl)
            n105 = Array Size(array=w406) -> (size(s)=w409:i32)
            n106 = Multiply(x=w409, y=w408) -> (x*y=w407:dbl)
            n107 = Bundle By Name(cluster=w401, "TestData"=0) -> (w399:T5)
            n108 = Round Toward -Infinity(1:w407) -> (0:w405:dbl)
            n109 = Index Array(array=w406, index=w405) -> (element=w404:string)
            n110 = call "CSM - Unregister Broadcast.vi"("CSM Name(Empty for Broadcast Event)"=w410, "Source CSM Name (* as Default)"=w404, "Trigger"="Test Status" ("Status"), "API (\"*\" as Default)"="Test State" ("Response Message (If \"\", Same as Source Message)")) -> ("error out"=w402:errorcluster)  [unwired: 10 in, 1 out]
            n111 = Merge Errors(w413, w402) -> (w403:errorcluster)
            n112 = call <vilib>:"Add State(s) to Queue__JKI_lib_State_Machine.vi"("State(s) in (\"\")"=w415) -> ("States Out"=w414:string)  [unwired: 14 in]
          }
        }
      }
      n113 = call "CSM - Wait for Module to Be Alive.vi"("CSM Name"=w6, "error in (no error)"=w7) -> ("error out"=w8:errorcluster)  [unwired: 11 in, 2 out]
      n114 = for {
        tunnel: w22 -> [w420] mode=indexing
        shift-right: [w419] -> w64
        shift-left: w8 -> [w418]
        n115 = call "uuid.vi"() -> ("UUID"=w421:string)  [unwired: 11 in]
        n116 = call "CSM - Wait and Send Message for Reply.vi"("State"="API: Test Register State", "Arguments (\"\")"=w421, "Target Module"=w420, "Wait (5000ms)"=60000, "Error In (No Error)"=w418) -> ("error out"=w419:errorcluster)  [unwired: 7 in, 3 out]
        n117 = Wait (ms)(milliseconds to wait=u32 2) -> ()  [unwired: 1 out]
      }
      n118 = Array Size(array=w22) -> (size(s)=w59:i32)
      n119 = call "Stall Data Flow.vim"("value in"=w64, "milliseconds to wait"=u32 100) -> ("value out"=w63:errorcluster)  [unwired: 1 out]
      n120 = call "CSM Get Module Attribute.vim"("CSM Name"=w6, "Attribute"=w55, "Default Value (Empty Variant)"=0 ("x+1"), "Error In"=w63) -> ("CSM Name (Dup)"=w56:string, "Found"=w61:bool, "Value"=w60:i32, "error out"=w54:errorcluster)  [unwired: 7 in, 1 out]
      n121 = Equal?(x=w59, y=w60) -> (x = y?=w58:bool)
      n122 = And(x=w61, y=w58) -> (x .and. y?=w57:bool)
      n123 = flat-sequence {
        tunnel: w56 -> [w93]
        tunnel: w55 -> [w92]
        tunnel: w54 -> [w91]
        tunnel: [w91] -> w53
        tunnel: [w90] -> w52
        tunnel: w6 -> [w98]
        tunnel: w53 -> [w97]
        tunnel: w52 -> [w96]
        tunnel: [w97] -> w51
        tunnel: [w96] -> w50
        tunnel: [w95] -> w49
        frame #0 {
          n124 = call "CSM - Delete Module Attribute.vi"("CSM Name"=w93, "Attribute"=w92) -> ("error out"=w90:errorcluster)  [unwired: 10 in, 3 out]
        }
        frame #1 {
          n125 = call "CSM - Wait and Send Message for Reply.vi"("State"="Unregister a random status", "Target Module"=w98, "Wait (5000ms)"=60000) -> ("error out"=w95:errorcluster)  [unwired: 9 in, 3 out]
        }
      }
      n126 = Merge Errors(w51, w50, w49) -> (w41:errorcluster)
      n127 = for {
        tunnel: w22 -> [w87] mode=indexing
        shift-right: [w86] -> w47
        shift-left: w41 -> [w85]
        n128 = call "uuid.vi"() -> ("UUID"=w88:string)  [unwired: 11 in]
        n129 = Wait (ms)(milliseconds to wait=u32 2) -> ()  [unwired: 1 out]
        n130 = call "CSM - Wait and Send Message for Reply.vi"("State"="API: Test Register State", "Arguments (\"\")"=w88, "Target Module"=w87, "Wait (5000ms)"=60000, "Error In (No Error)"=w85) -> ("error out"=w86:errorcluster)  [unwired: 7 in, 3 out]
      }
      n131 = Array Size(array=w22) -> (size(s)=w40:i32)
      n132 = Decrement(x=w40) -> (x-1=w39:i32)
      n133 = call "Stall Data Flow.vim"("value in"=w47, "milliseconds to wait"=u32 100) -> ("value out"=w46:errorcluster)  [unwired: 1 out]
      n134 = call "CSM Get Module Attribute.vim"("CSM Name"=w6, "Attribute"=w33, "Default Value (Empty Variant)"=0 ("x+1"), "Error In"=w46) -> ("CSM Name (Dup)"=w34:string, "Found"=w44:bool, "Value"=w43:i32, "error out"=w32:errorcluster)  [unwired: 7 in, 1 out]
      n135 = Equal?(x=w39, y=w43) -> (x = y?=w42:bool)
      n136 = And(x=w44, y=w42) -> (x .and. y?=w28:bool)
      n137 = flat-sequence {
        tunnel: w34 -> [w75]
        tunnel: w33 -> [w74]
        tunnel: w32 -> [w73]
        tunnel: [w73] -> w36
        tunnel: [w72] -> w35
        tunnel: w6 -> [w81]
        tunnel: w36 -> [w80]
        tunnel: w35 -> [w79]
        tunnel: [w80] -> w31
        tunnel: [w79] -> w30
        tunnel: [w77] -> w29
        frame #0 {
          n138 = call "CSM - Delete Module Attribute.vi"("CSM Name"=w75, "Attribute"=w74) -> ("error out"=w72:errorcluster)  [unwired: 10 in, 3 out]
        }
        frame #1 {
          n139 = call "CSM - Wait and Send Message for Reply.vi"("State"="Macro: Exit", "Target Module"=w81, "Response Timeout (-2 Using Global Settings)"=60000) -> ("error out"=w78:errorcluster)  [unwired: 9 in, 3 out]
          n140 = call <vilib>:"Clear Errors.vi"("error in (no error)"=w78) -> ("error out"=w77:errorcluster)  [unwired: 5 in, 1 out]
        }
      }
      n141 = Merge Errors(w31, w30, w29) -> (w12:errorcluster)
      n142 = call "Package Error Info.vi"("error in"=w12, "String in"="General Error") -> ("packed error info out"=w13:string, "error status"=w17:bool)  [unwired: 8 in]
      n143 = call-dynamic "failIf.vi"("message (\"\")"=w13, "fail"=w17, "TestCase in"=w16) -> ("error out"=w14:errorcluster, "TestCase out"=w15:refnum<class "testcase-CSMBroadcast.lvclass">)  [unwired: 7 in]
      n144 = call-dynamic "passIf.vi"("error in (no error)"=w14, "message (\"\")"="Before unreigster" ("message (\"\")"), "pass"=w57, "TestCase in"=w15) -> ("error out"=w38:errorcluster, "TestCase out"=w37:refnum<class "testcase-CSMBroadcast.lvclass">)  [unwired: 6 in]
      n145 = call-dynamic "passIf.vi"("error in (no error)"=w38, "message (\"\")"="After unregister" ("message (\"\")"), "pass"=w28, "TestCase in"=w37) -> ("error out"=w20:errorcluster, "TestCase out"=w21:refnum<class "testcase-CSMBroadcast.lvclass">)  [unwired: 6 in]
      n146 = flat-sequence {
        tunnel: w20 -> [w71]
        tunnel: [w70] -> w18
        tunnel: w21 -> [w68]
        tunnel: [w68] -> w19
        frame #0 {
          n147 = call "CSM - Drop Broadcast Registry.vi"() -> ("error out"=w69:errorcluster)  [unwired: 15 in]
          n148 = Merge Errors(w71, w69) -> (w70:errorcluster)
        }
      }
    }
    frame Disabled {
      # "skip test result while test is under development"
      n149 = call <vilib>:"skip.vi"("error in (no error)"=w423, "TestCase in"=w426) -> ("error out"=w425:errorcluster, "TestCase out"=w424:refnum<class "testcase-CSMBroadcast.lvclass">)  [unwired: 8 in]
    }
  }
  "error out" <- w4
  "TestCase out" <- w2
